vi "Expression Format Example.vi"() -> ()   [LabVIEW 2017, in "Logger Examples.lvlib"]
uses:
  Logger Examples.lvlib
  Source/Composed Log/Types/Log Level.ctl
  Source/String Formats/String Expression Format/String Expression Format.lvclass/String Expression Format.ctl
  Source/Composed Log/LoggerReference/LoggerReference.lvclass/LoggerReference.ctl
  601d143e-8928-4a3b-9174-3083e729aaa9.vi
  Source/String Formats/String Expression Format/Run Formatter.vi
  Source/Composed Log/LoggerReference/Return Aggregate Queues.vi
  Source/Composed Log/LoggerReference/Add Aggregate Log.vi
  601d143e-8928-4a3b-9174-3083e729aaa9.vi/206ceb10-35a2-4605-9eb4-9c8c591005a9.vi
  Source/Composed Log/LoggerReference/Log.vi
  Source/Composed Log/LoggerReference/Get Valid Event Time.vi
  <vilib>/dlg_ctls.llb/Space Constant.vi
  Source/Composed Log/LoggerReference/Send Add Sink.vi
  Source/Composed Log/LoggerReference/Remove Stale Logs.vi
  Source/String Formats/String Expression Format/String Expression Format.lvclass
  C:/CS/Internal/LabVIEW/Logger/Source/IStringFormat/IStringFormat.lvclass
  Source/String Control Sink/String Control Sink.lvclass
  C:/CS/Internal/LabVIEW/Logger/Source/Composed Log/Log Sink/Log Sink.lvclass
  Source/Composed Log/Application Logger/Launch Worker Loop.vi
  Source/Composed Log/LoggerReference/Initialize Logger Instance.vi
  Source/Composed Log/LoggerReference/LoggerReference.lvclass
  Source/Composed Log/IErrorFormat/IErrorFormat.lvclass
  Source/Composed Log/Log Sink/Log Sink.lvclass
  Source/Composed Log/Composed Log.lvlib
panel:
  in  "Log Error":bool
  in  "Error Information":string
  in  "Error Code":i32
  in  "Event Level":T1(ring)
  out "Event - %s[EVT]  - Occured at <%T>[TIME] From %s[ID], Level %s[LVL]":string
  out "%<%A at %H:%M:%S>T[TIME] -- %s[EVT]":string
  out "<%T>[TIME]<%s[LVL]-%s[ID]><%s>[EVT]":string
  in  "Data To Log":string
  in  "Source":string="User"
  in  "Log":bool
  # "Run the VI. Note the different formats - each string indicator is displaying the same event with different string format."
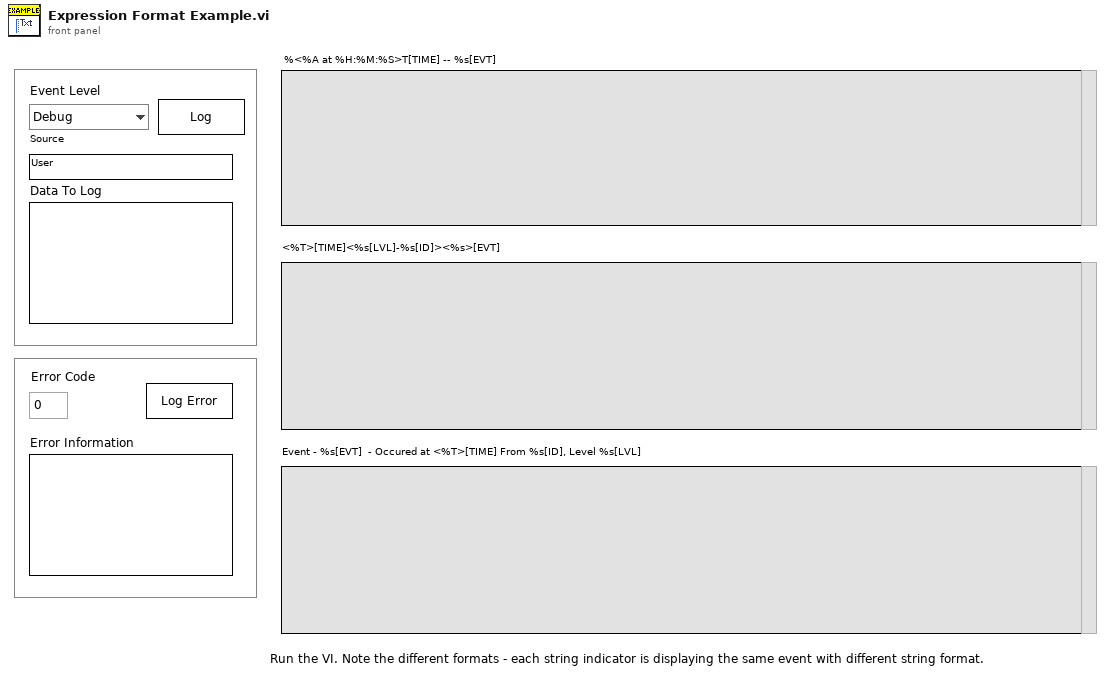
[diagram p1: front panel]
types:
  T1 = enum16{"Debug", "Info", "Warning", "Error", "Critical"}
  T2 = typedef "Composed Log.lvlib/Log Level.ctl" = enum16{"Debug", "Info", "Warning", "Error", "Critical"}
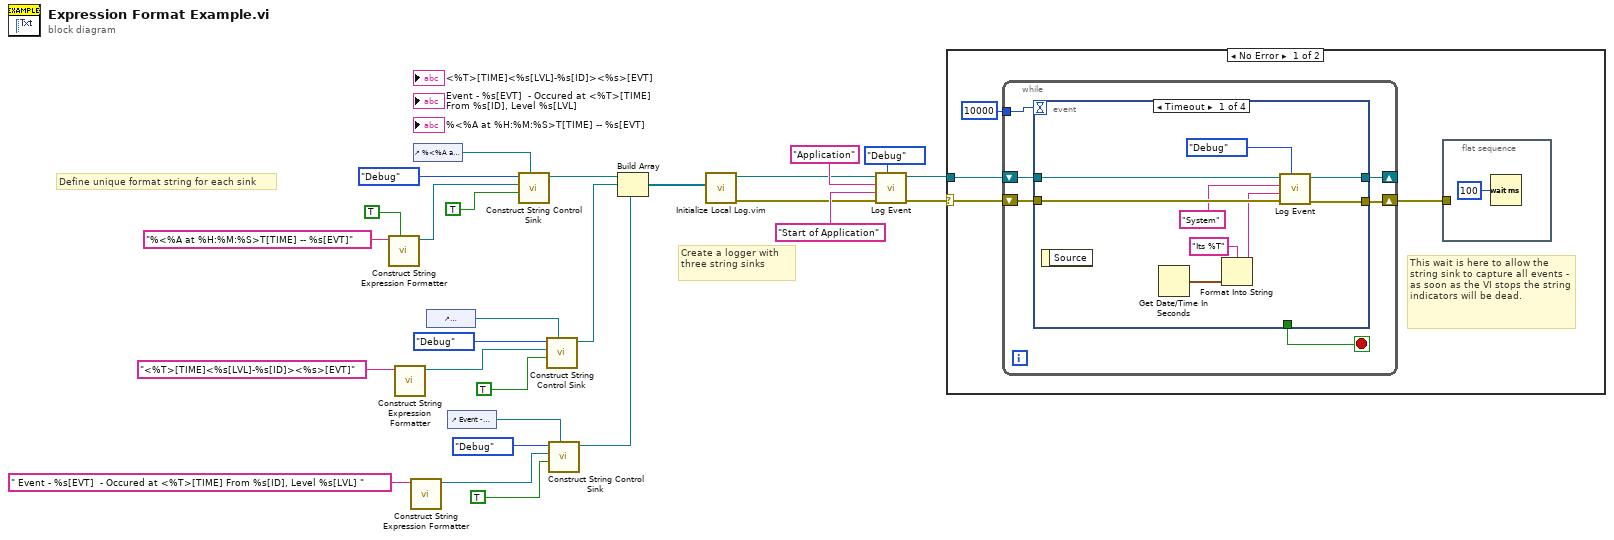
[diagram p0: block diagram]
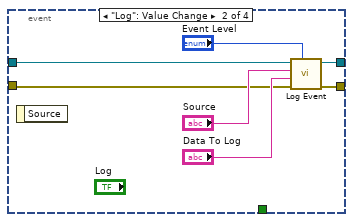
[diagram p2: hidden frame]
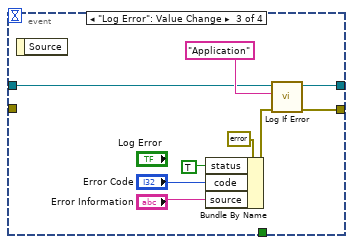
[diagram p3: hidden frame]
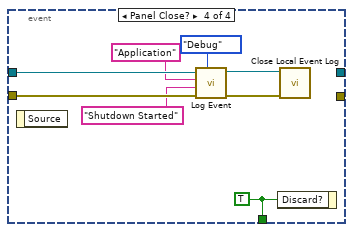
[diagram p4: hidden frame]
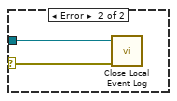
[diagram p5: hidden frame]
diagram:
  # "Define unique format string for each sink"
  # "Create a logger with three string sinks"
  n1 = call "Construct String Expression Formatter.vi"("Append EOL?"=TRUE, "Format Specifier"="%<%A at %H:%M:%S>T[TIME] -- %s[EVT]") -> ("String Expression Format out"=w10:refnum<class "String Expression Format.lvclass">)  [unwired: 8 in, 1 out]
  n2 = call "Construct String Expression Formatter.vi"("Format Specifier"="<%T>[TIME]<%s[LVL]-%s[ID]><%s>[EVT]") -> ("String Expression Format out"=w7:refnum<class "String Expression Format.lvclass">)  [unwired: 9 in, 1 out]
  n3 = call "Construct String Expression Formatter.vi"("Format Specifier"=" Event - %s[EVT]  - Occured at <%T>[TIME] From %s[ID], Level %s[LVL] ") -> ("String Expression Format out"=w3:refnum<class "String Expression Format.lvclass">)  [unwired: 9 in, 1 out]
  n4 = control-ref of="%<%A at %H:%M:%S>T[TIME] -- %s[EVT]"() -> (w23:refnum<vi>)
  n5 = control-ref of="<%T>[TIME]<%s[LVL]-%s[ID]><%s>[EVT]"() -> (w25:refnum<vi>)
  n6 = control-ref of="Event - %s[EVT]  - Occured at <%T>[TIME] From %s[ID], Level %s[LVL]"() -> (w19:refnum<vi>)
  n7 = call "Construct String Control Sink.vi"("Str Refnum"=w23, "AutoScroll?(F)"=TRUE, "LogFormat"=w10, "LogLevel"=Log_Level."Debug") -> ("String Control Sink out"=w18:refnum<class "String Control Sink.lvclass">)  [unwired: 7 in]
  n8 = call "Construct String Control Sink.vi"("Str Refnum"=w25, "AutoScroll?(F)"=TRUE, "LogFormat"=w7, "LogLevel"=Log_Level."Debug") -> ("String Control Sink out"=w6:refnum<class "String Control Sink.lvclass">)  [unwired: 7 in]
  n9 = call "Construct String Control Sink.vi"("Str Refnum"=w19, "AutoScroll?(F)"=TRUE, "LogFormat"=w3, "LogLevel"=Log_Level."Debug") -> ("String Control Sink out"=w2:refnum<class "String Control Sink.lvclass">)  [unwired: 7 in]
  n10 = Build Array(w18, w6, w2) -> (w1:refnum<class "String Control Sink.lvclass">[])
  n11 = call "Initialize Local Log.vim"("Startup Sink(s)"=w1) -> ("error out"=w14:errorcluster, "Log Instance Reference"=w13:refnum<class "LoggerReference.lvclass">)  [unwired: 8 in, 1 out]
  n12 = call "Log Event.vi"("Event Level"=Log_Level."Debug", "error in (no error)"=w14, "Data To Log"="Start of Application", "SourceID"="Application", "Log Instance"=w13) -> ("error out"=w12:errorcluster, "Log Instance Out"=w11:refnum<class "LoggerReference.lvclass">)  [unwired: 5 in]
  n13 = case shown="No Error" w12 {
    selector: w12 -> [w30 w72]
    tunnel: w11 -> [w31 w73]
    frame No Error {
      # "This wait is here to allow the string sink to capture all events - as soon as the VI stops the string indicators will be dead."
      n14 = while {
        shift-right: [w36] -> _
        shift-left: w31 -> [w37]
        shift-right: [w34] -> w28
        shift-left: w30 -> [w35]
        tunnel: 10000 -> [w33]
        stop <- w38 stop-if-true
        n15 = event shown="[0] Timeout" {
          selector: _ -> [_ _ _ _]
          dyn-events: _ -> [_ _ _ _]
          timeout: w33 -> [_ _ _ _]
          tunnel: [_ _ _ w71] -> w38
          tunnel: w37 -> [w47 w51 w57 w69]
          tunnel: [w46 w49 w55 _] -> w36
          tunnel: w35 -> [w44 w48 _ w70]
          tunnel: [w43 w50 w56 _] -> w34
          event Timeout {
            n16 = event-data() -> ()  [unwired: 1 in, 1 out]
            n17 = Get Date/Time In Seconds() -> (seconds since 1Jan1904=w41:timestamp)
            n18 = Format Into String(format string="Its %T" ("Log Message"), w41) -> (resulting string=w39:string)  [unwired: 2 in, 1 out]
            n19 = call "Log Event.vi"("Event Level"=Log_Level."Debug", "error in (no error)"=w44, "Data To Log"=w39, "SourceID"="System" ("Event Source"), "Log Instance"=w47) -> ("error out"=w43:errorcluster, "Log Instance Out"=w46:refnum<class "LoggerReference.lvclass">)  [unwired: 5 in]
          }
          event "Log": Value Change {
            n20 = event-data() -> ()  [unwired: 1 in, 1 out]
            n21 = call "Log Event.vi"("Event Level"="Event Level", "error in (no error)"=w48, "Data To Log"="Data To Log", "SourceID"="Source", "Log Instance"=w51) -> ("error out"=w50:errorcluster, "Log Instance Out"=w49:refnum<class "LoggerReference.lvclass">)  [unwired: 5 in]
          }
          event "Log Error": Value Change {
            n22 = event-data() -> ()  [unwired: 1 in, 1 out]
            n23 = Bundle By Name(cluster=errorcluster {"status"=FALSE, "code"=0, "source"=""} ("Error In"), "status"=TRUE, "code"="Error Code", "source"="Error Information") -> (w61:errorcluster)
            n24 = call "Log If Error.vi"("Error In"=w61, "SourceID"="Application" ("Source"), "Log Instance"=w57) -> ("error out"=w56:errorcluster, "Log Instance Out"=w55:refnum<class "LoggerReference.lvclass">)  [unwired: 7 in]
          }
          event Panel Close? {
            w71 = TRUE ("Discard?")
            n25 = event-data() -> ()  [unwired: 1 in, 1 out]
            n26 = call "Log Event.vi"("Event Level"=Log_Level."Debug", "error in (no error)"=w70, "Data To Log"="Shutdown Started", "SourceID"="Application", "Log Instance"=w69) -> ("error out"=w68:errorcluster, "Log Instance Out"=w67:refnum<class "LoggerReference.lvclass">)  [unwired: 5 in]
            n27 = event-data("Discard?"=w71) -> ()  [unwired: 1 in, 1 out]
            n28 = call "Close Local Event Log.vi"("error in (no error)"=w68, "Log Instance"=w67) -> ()  [unwired: 9 in, 1 out]
          }
        }
      }
      n29 = flat-sequence {
        tunnel: w28 -> [_]
        frame #0 {
          n30 = Wait (ms)(milliseconds to wait=u32 100) -> ()  [unwired: 1 out]
        }
      }
    }
    frame Error {
      n31 = call "Close Local Event Log.vi"("error in (no error)"=w72, "Log Instance"=w73) -> ()  [unwired: 9 in, 1 out]
    }
  }
